vi "DialogRenameVI.vi"(0 "ClassWriter.lvclass":refnum<class "ClassWriter.lvclass">, 1 "VIItemRefIn":refnum<vi>, 5 "error in (no error)":errorcluster) -> (14 "ClassWriter.lvclassOut":refnum<class "ClassWriter.lvclass">, 15 "Cancelled":bool, 16 "RenameOption":T1, 19 "error out":errorcluster)   [LabVIEW 2020, in "ClassWriter.lvclass"]
uses:
  <resource>/Framework/Providers/Open_GDS/ClassProviders/Provider_BaseClassInterface/ClassWriter_class/ClassWriter.lvclass
  <resource>/Framework/Providers/Open_GDS/ClassProviders/Provider_BaseClassInterface/ClassWriter_class/RenameViOption.ctl
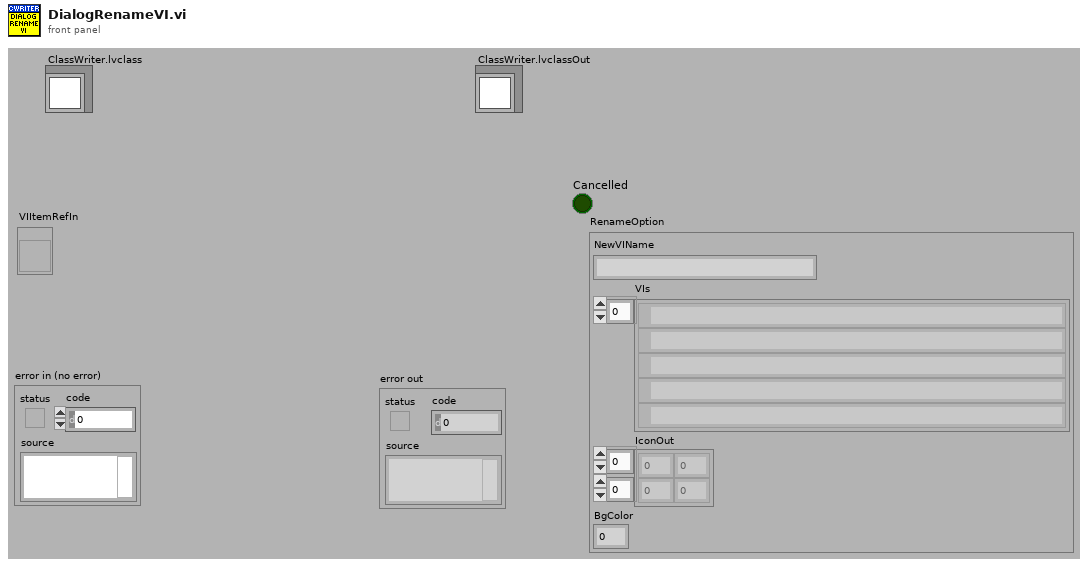
[diagram p1: front panel]
types:
  T1 = typedef "ClassWriter.lvclass/RenameViOption.ctl" = cluster{"NewVIName":string, "VIs":path[], "IconOut":u8[][], "BgColor":u8}
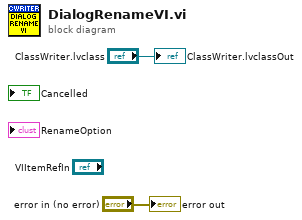
[diagram p0: block diagram]
diagram:
  "error out" <- "error in (no error)"
  "ClassWriter.lvclassOut" <- "ClassWriter.lvclass"
